vi "GetConfig.vi"(8 "error in (no error)":errorcluster, 11 "PmuTestFunctions in":refnum<class "PmuTestFunctions.lvclass">) -> (0 "error out":errorcluster, 2 "Config":variant, 3 "PmuTestFunctions out":refnum<class "PmuTestFunctions.lvclass">)   [LabVIEW 2014, in "Functions.lvlib" / "PmuTestFunctions.lvclass"]
uses:
  PmuTestFunctions.lvclass
  PmuTestConfig.ctl
  ArbitraryFunction/TypeDefs/ArbCfg.ctl
  ArbitraryFunction/TypeDefs/Arbitrary.ctl
  PmuTestFunctions.lvclass/PmuTestFunctions.ctl
  Accessors/Read T0.vi
  Accessors/Read SettlingTime.vi
  ArbitraryFunction/ArbitraryFunction.lvclass
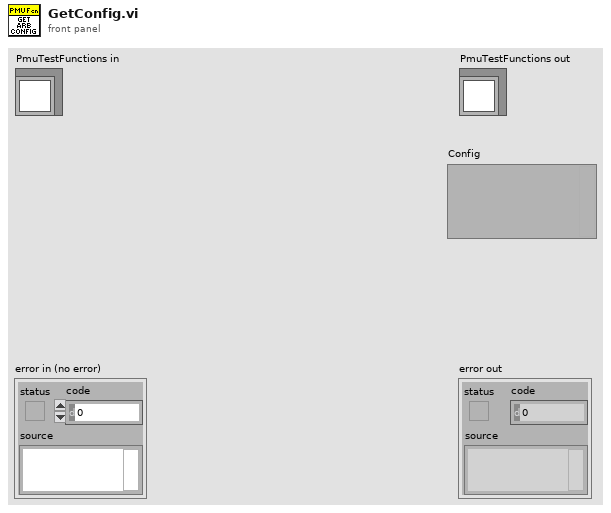
[diagram p1: front panel]
types:
  T1 = typedef "Functions.lvlib/ArbitraryFunction.lvclass/ArbCfg.ctl" = cluster{"SampleRate":dbl, "Count":u16, "Arbs":T2[]}
  T2 = typedef "Functions.lvlib/ArbitraryFunction.lvclass/Arbitrary.ctl" = cluster{"Handle":string, "Size":i32, "Gain":dbl, "Offset":dbl, "Waveform":waveform(dbl)}
  T3 = typedef "Functions.lvlib/PmuTestFunctions.lvclass/PmuTestConfig.ctl" = cluster{"T0":dbl, "SettlingTime":dbl, "ArbCfg":T1}
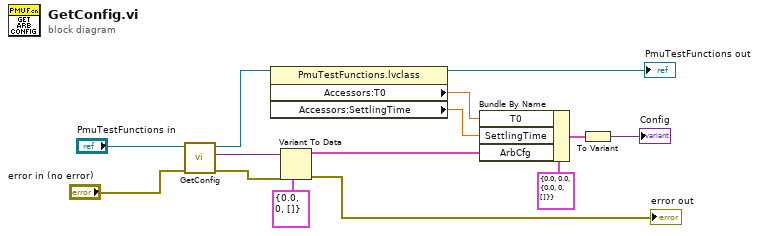
[diagram p0: block diagram]
diagram:
  n1 = call-parent "GetConfig.vi"("error in (no error)"="error in (no error)", "ArbitraryFunction in"="PmuTestFunctions in") -> ("error out"=w4:errorcluster, "Config"=w5:variant, "ArbitraryFunction out"=w14:refnum<class "PmuTestFunctions.lvclass">)  [unwired: 7 in]
  n2 = property class="PmuTestFunctions.lvclass"(reference=w14) -> (reference out=→"PmuTestFunctions out":refnum<class "PmuTestFunctions.lvclass">, "Accessors:T0"=w9:dbl, "Accessors:SettlingTime"=w8:dbl)  [unwired: 1 in, 1 out]
  n3 = Variant To Data(error in=w4, type=T1 {"SampleRate"=0.0, "Count"=0, "Arbs"=[]} ("ArbCfg"), Variant=w5) -> (data=w1:T1, error out=→"error out":errorcluster)
  n4 = Bundle By Name(cluster=T3 {"T0"=0.0, "SettlingTime"=0.0, "ArbCfg"={"SampleRate"=0.0, "Count"=0, "Arbs"=[]}} ("PmuTestConfig"), "T0"=w9, "SettlingTime"=w8, "ArbCfg"=w1) -> (w7:T3)
  n5 = To Variant(anything=w7) -> (Variant=→"Config":variant)
